vi "InitializeStageOutput.vi"(2 "Image Settings":T1={"Start Position (µm)"={"x"=0.0, "y"=0.0, "z"=0.0}, "End Position (µm)"={"x"=10.0, "y"=10.0, "z"=0.0}, "Image Resolution (nm/pixel)"={"x"=50.0, "y"=50.0, "z"=100.0}, "Image Size (µm)"={"x"=10.0, "y"=10.0, "z"=0.0}, "Image Size (pixel)"={"x"=50, "y"=50, "z"=0}, "Time Resolution\n(ms/pixel)"=7.0, "1st Axis"=0, "2nd Axis"=1, "Retrace"=FALSE, "Estimated Time"=""} {"2nd Axis" items=["x", "y", "z"]; "1st Axis" items=["x", "y", "z"]; "Time Resolution\n(ms/pixel)" format="%.2f"; "Image Resolution (nm/pixel)"."z" format="%.2f"; "Image Resolution (nm/pixel)"."y" format="%.2f"; "Image Resolution (nm/pixel)"."x" format="%.2f"; "Image Size (µm)"."z" format="%.2f"; "Image Size (µm)"."y" format="%.2f"; "Image Size (µm)"."x" format="%.2f"; "End Position (µm)"."z" format="%.2f"; "End Position (µm)"."y" format="%.2f"; "End Position (µm)"."x" format="%.2f"; "Start Position (µm)"."z" format="%.2f"; "Start Position (µm)"."y" format="%.2f"; "Start Position (µm)"."x" format="%.2f"}, 3 "Timing Info":T2 {"#s" format="%.2f"; "Fs" format="%.2f"}) -> (0 "Error out":errorcluster, 1 "Analog Output":T3)   [LabVIEW 2009]
uses:
  AnalogTrace.ctt
  TimingInfo.ctt
  ImageSettings.ctt
panel:
  in  "VI Refnum":refnum<vi>
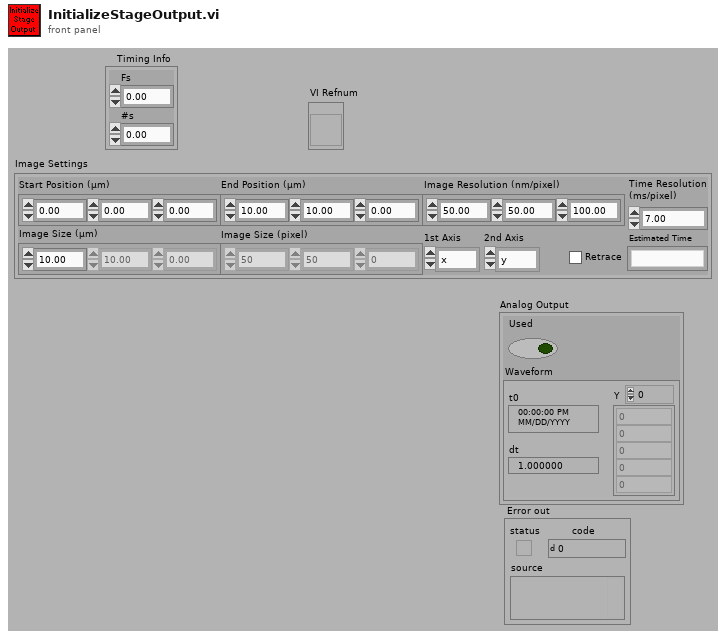
[diagram p1: front panel]
types:
  T1 = typedef "ImageSettings.ctt" = cluster{"Start Position (µm)":cluster{"x":dbl, "y":dbl, "z":dbl}, "End Position (µm)":cluster{"x":dbl, "y":dbl, "z":dbl}, "Image Resolution (nm/pixel)":cluster{"x":dbl, "y":dbl, "z":dbl}, "Image Size (µm)":cluster{"x":dbl, "y":dbl, "z":dbl}, "Image Size (pixel)":cluster{"x":u32, "y":u32, "z":u32}, "Time Resolution\n(ms/pixel)":dbl, "1st Axis":u16, "2nd Axis":u16, "Retrace":bool, "Estimated Time":string}
  T2 = typedef "TimingInfo.ctt" = cluster{"Fs":dbl, "#s":dbl}
  T3 = typedef "AnalogTrace.ctt" = cluster{"Used":bool, "Waveform":waveform(dbl)}
  T4 = enum16{"Get Type", "Set Type", "GetStageInit", "GetWriteStageSetting", "GetInitializeStageOutput", "GetSetAxisPosition", "GetSetPos"}
  T5 = typedef "StageType.ctt" = enum16{"PI 725 USB", "PI 725 TCP/IP", "PI analogue step"}
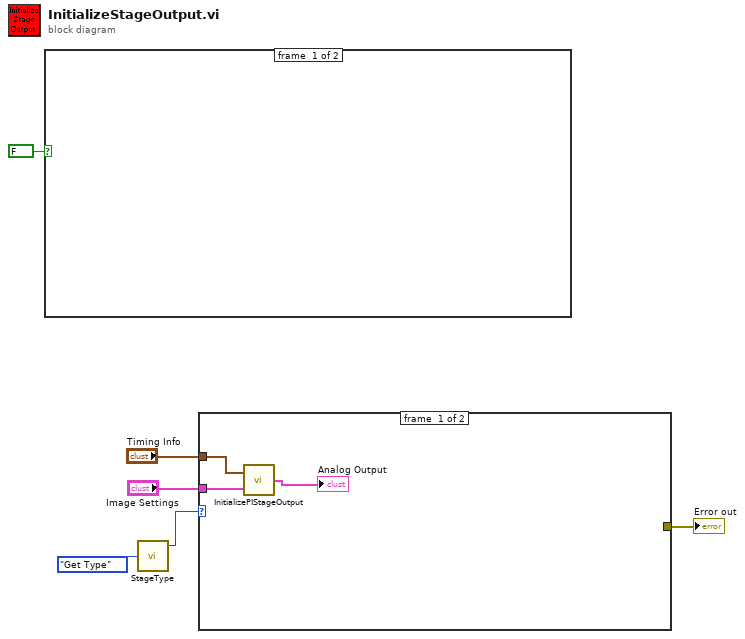
[diagram p0: block diagram]
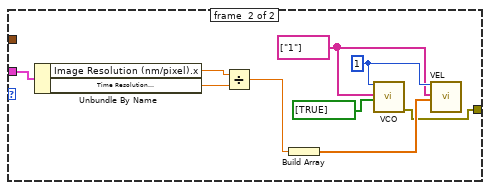
[diagram p2: hidden frame]
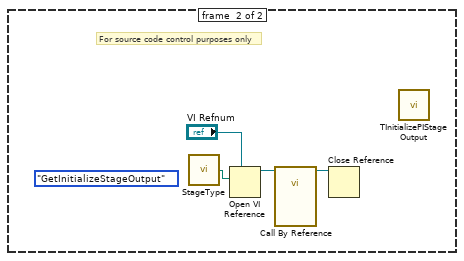
[diagram p3: hidden frame]
diagram:
  n1 = case shown="False" FALSE ("Case Constant\n(See Context Help)") {
    frame #0 {
    }
    frame #1 {
      (unwired) T4."GetInitializeStageOutput" ("Function")
      # "For source code control purposes only"
      n2 = call "StageType.vi"() -> ("VI Path"=w7:path)  [unwired: 3 in, 2 out]
      n3 = Open VI Reference(type specifier VI Refnum (for type only)="VI Refnum", vi path=w7) -> (vi reference=w8:refnum<vi>)  [unwired: 4 in, 1 out]
      n4 = call-by-ref "?"(reference=w8) -> (reference out=w9:refnum<vi>)  [unwired: 3 in, 2 out]
      n5 = Close Reference(reference=w9) -> ()  [unwired: 1 in, 1 out]
      n6 = call "TInitializePIStageOutput.vi"() -> ()  [unwired: 2 in, 1 out]
    }
  }
  n7 = call "StageType.vi"("Function"=T4."Get Type") -> ("Stage Type (output)"=w2:T5)  [unwired: 2 in, 2 out]
  n8 = case shown="\"PI 725 USB\", \"PI 725 TCP/IP\"" w2 {
    tunnel: "Timing Info" -> [w13 _]
    tunnel: "Image Settings" -> [w12 w19]
    tunnel: [_ w15] -> w1
    frame #0 {
      n9 = call "InitializePIStageOutput.vi"("Image Settings"=w12, "Timing Info"=w13) -> ("Analog Output"=→"Analog Output":T3)
    }
    frame #1 {
      w21 = string[] ["1"] ("Axes to command")
      w22 = 1 ("System no.")
      n10 = Unbundle By Name(w19) -> ("Image Resolution (nm/pixel).x"=w18:dbl, "Time Resolution\n(ms/pixel)"=w17:dbl)
      n11 = Divide(x=w18, y=w17) -> (x/y=w14:dbl)
      n12 = Build Array(w14) -> (w16:dbl[])
      n13 = call "VCO.vi"("System no."=w22, "Axes to command"=w21, "Vel. control mode"=bool[] [TRUE]) -> ("error out"=w15:errorcluster)  [unwired: 16 in]
      n14 = call "VEL.vi"("System no."=w22, "Axes to set"=w21, "Velocity values"=w16) -> ()  [unwired: 15 in, 2 out]
    }
  }
  "Error out" <- w1
